vi "Global 4.vi"() -> ()   [LabVIEW 2016]
panel:
  in  "Stop Button":bool
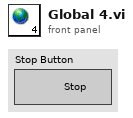
[diagram p1: front panel]
diagram:
